vi "RichToFlatnixnet_grpc_WaitRequest.vi"(5 "OutputClusterType":T1, 11 "InputCluster":T4) -> (3 "OutputCluster":T1)   [LabVIEW 2025, in "grpc-xnet_client.lvlib"]
uses:
  grpc-xnet_client.lvlib
  nixnet_grpc_WaitRequest.ctl
  nixnet_grpc_WaitRequest_condition_enum/nixnet_grpc_WaitRequest_condition_enum.lvclass
  nidevice_grpc_Session.ctl
  nixnet_grpc_WaitRequest_Flat.ctl
  nidevice_grpc_Session_Flat.ctl
  nixnet_grpc_WaitCondition.ctl
  nixnet_grpc_WaitRequest_condition_enum/nixnet_grpc_WaitRequest_condition_enum.lvclass/nixnet_grpc_WaitRequest_condition_enum.ctl
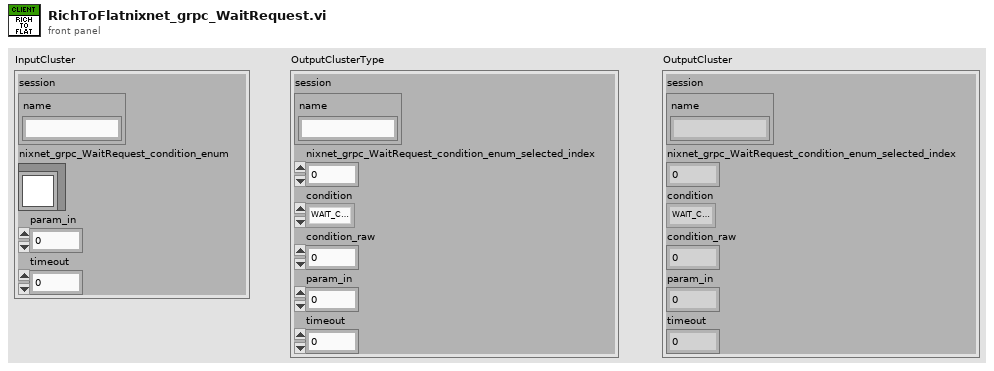
[diagram p1: front panel]
types:
  T1 = typedef "grpc-xnet_client.lvlib/nixnet_grpc_WaitRequest_Flat.ctl" = cluster{"session":T2, "nixnet_grpc_WaitRequest_condition_enum_selected_index":i32, "condition":T3, "condition_raw":u32, "param_in":u32, "timeout":dbl}
  T2 = typedef "grpc-xnet_client.lvlib/nidevice_grpc_Session_Flat.ctl" = cluster{"name":string}
  T3 = typedef "grpc-xnet_client.lvlib/nixnet_grpc_WaitCondition.ctl" = enum32{"WAIT_CONDITION_UNSPECIFIED", "WAIT_CONDITION_TRANSMIT_COMPLETE", "WAIT_CONDITION_INTF_COMMUNICATING", "WAIT_CONDITION_INTF_REMOTE_WAKEUP", "WAIT_CONDITION_ETHERNET_SYNCED"}
  T4 = typedef "grpc-xnet_client.lvlib/nixnet_grpc_WaitRequest.ctl" = cluster{"session":T5, "nixnet_grpc_WaitRequest_condition_enum":refnum<class "nixnet_grpc_WaitRequest_condition_enum.lvclass">, "param_in":u32, "timeout":dbl}
  T5 = typedef "grpc-xnet_client.lvlib/nidevice_grpc_Session.ctl" = cluster{"name":string}
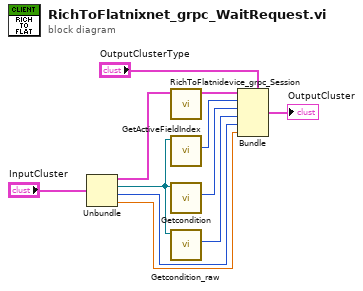
[diagram p0: block diagram]
diagram:
  n1 = Unbundle "Unbundle"("InputCluster") -> ("session"=w8:T5, "nixnet_grpc_WaitRequest_condition_enum"=w6:refnum<class "nixnet_grpc_WaitRequest_condition_enum.lvclass">, "param_in"=w2:u32, "timeout"=w1:dbl)
  n2 = call "RichToFlatnidevice_grpc_Session.vi"("InputCluster"=w8) -> ("OutputCluster"=w7:T2)  [unwired: 10 in]
  n3 = call "GetActiveFieldIndex.vi"("OneOfTemplate in"=w6) -> ("Active Field Index"=w5:i32)  [unwired: 8 in, 2 out]
  n4 = call "Getcondition.vi"("OneOfTemplate in"=w6) -> ("Get_Val"=w4:T3)  [unwired: 8 in, 2 out]
  n5 = call "Getcondition_raw.vi"("OneOfTemplate in"=w6) -> ("Get_Val"=w3:u32)  [unwired: 8 in, 2 out]
  n6 = Bundle "Bundle"(cluster="OutputClusterType", "session"=w7, "nixnet_grpc_WaitRequest_condition_enum_selected_index"=w5, "condition"=w4, "condition_raw"=w3, "param_in"=w2, "timeout"=w1) -> (→"OutputCluster":T1)
